vi "OP300ZP_prep bdd datadyn.vi"(8 "tabin":string[](array[string]), 11 "StrData":T1={"Chaîne"="20.0", "Chaîne"="22.0", "Chaîne"="3560", "Chaîne"="3561", "Chaîne"="25.0", "Chaîne"="2.0", "Chaîne"=" 1.0", "Chaîne 2"=" 1.0"}) -> (0 "tabout":string[](array[string]))   [LabVIEW 2020]
uses:
  OP300ZP_selectdata.ctl
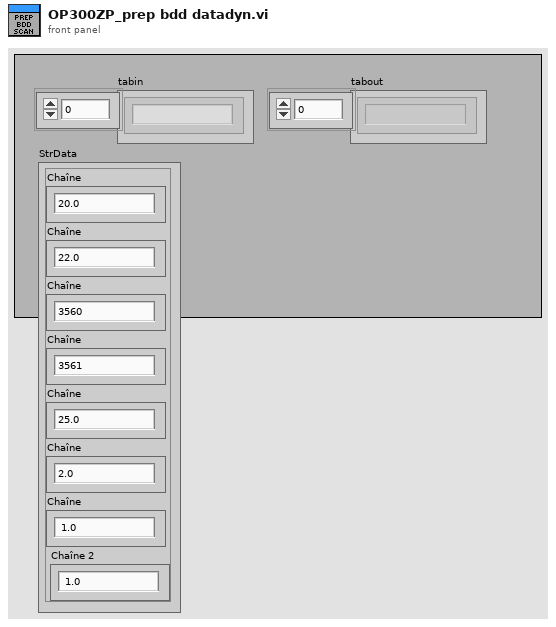
[diagram p1: front panel]
types:
  T1 = cluster{"Chaîne":string, "Chaîne":string, "Chaîne":string, "Chaîne":string, "Chaîne":string, "Chaîne":string, "Chaîne":string, "Chaîne 2":string}
  T2 = typedef "OP300ZP_selectdata.ctl" = u16
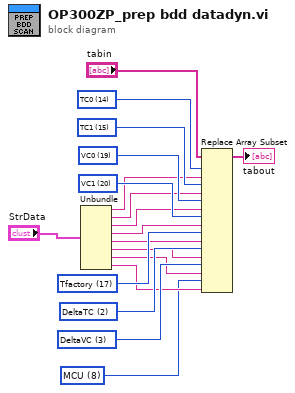
[diagram p0: block diagram]
diagram:
  w1 = T2 8 items=["IdOp300", "DateStart", "DeltaTC", "DeltaVC", "ImageVers", "IniFileVers", "InsuN", "InsuP", "MCU", "OCV", "Operateur", "Pass", "SN", "SoftVers", "TC0", "TC1", "TempsTest", "Tfactory", "Type", "VC0", "VC1"] ("Menu déroulant")
  w12 = T2 3 items=["IdOp300", "DateStart", "DeltaTC", "DeltaVC", "ImageVers", "IniFileVers", "InsuN", "InsuP", "MCU", "OCV", "Operateur", "Pass", "SN", "SoftVers", "TC0", "TC1", "TempsTest", "Tfactory", "Type", "VC0", "VC1"] ("Menu déroulant")
  w13 = T2 2 items=["IdOp300", "DateStart", "DeltaTC", "DeltaVC", "ImageVers", "IniFileVers", "InsuN", "InsuP", "MCU", "OCV", "Operateur", "Pass", "SN", "SoftVers", "TC0", "TC1", "TempsTest", "Tfactory", "Type", "VC0", "VC1"] ("Menu déroulant")
  w14 = T2 17 items=["IdOp300", "DateStart", "DeltaTC", "DeltaVC", "ImageVers", "IniFileVers", "InsuN", "InsuP", "MCU", "OCV", "Operateur", "Pass", "SN", "SoftVers", "TC0", "TC1", "TempsTest", "Tfactory", "Type", "VC0", "VC1"] ("Menu déroulant")
  w15 = T2 20 items=["IdOp300", "DateStart", "DeltaTC", "DeltaVC", "ImageVers", "IniFileVers", "InsuN", "InsuP", "MCU", "OCV", "Operateur", "Pass", "SN", "SoftVers", "TC0", "TC1", "TempsTest", "Tfactory", "Type", "VC0", "VC1"] ("Menu déroulant")
  w16 = T2 19 items=["IdOp300", "DateStart", "DeltaTC", "DeltaVC", "ImageVers", "IniFileVers", "InsuN", "InsuP", "MCU", "OCV", "Operateur", "Pass", "SN", "SoftVers", "TC0", "TC1", "TempsTest", "Tfactory", "Type", "VC0", "VC1"] ("Menu déroulant")
  w17 = T2 15 items=["IdOp300", "DateStart", "DeltaTC", "DeltaVC", "ImageVers", "IniFileVers", "InsuN", "InsuP", "MCU", "OCV", "Operateur", "Pass", "SN", "SoftVers", "TC0", "TC1", "TempsTest", "Tfactory", "Type", "VC0", "VC1"] ("Menu déroulant")
  w18 = T2 14 items=["IdOp300", "DateStart", "DeltaTC", "DeltaVC", "ImageVers", "IniFileVers", "InsuN", "InsuP", "MCU", "OCV", "Operateur", "Pass", "SN", "SoftVers", "TC0", "TC1", "TempsTest", "Tfactory", "Type", "VC0", "VC1"] ("Menu déroulant")
  n1 = Unbundle("StrData") -> ("Chaîne"=w10:string, "Chaîne"=w8:string, "Chaîne"=w7:string, "Chaîne"=w6:string, "Chaîne"=w5:string, "Chaîne"=w4:string, "Chaîne"=w3:string, "Chaîne 2"=w2:string)
  n2 = Replace Array Subset(array="tabin", new element #1=w10, index #1=w18, new element #2=w8, index #2=w17, new element #3=w7, index #3=w16, new element #4=w6, index #4=w15, new element #5=w5, index #5=w14, new element #6=w4, index #6=w13, new element #7=w3, index #7=w12, new element #8=w2, index #8=w1) -> (→"tabout":string[])
